vi "Add Channel to Objects.vi"(8 "error in":errorcluster, 9 "Add? (T)":bool=TRUE, 10 "Line Item in":T1, 11 "Objects in":T4) -> (0 "error out":errorcluster, 2 "Line Index":i32)   [LabVIEW 2013, in "FPGA Module editor node.lvclass"]
doc: "This VI adds the channel to the configuration Objects, and links the tag and the channel in the engine."
uses:
  FPGA Module editor node.lvclass
  <vilib>/NI/DCAF/Tag Editor Core/Table API/Table Manager/object ref.ctl
  <vilib>/NI/DCAF/Tag Editor Core/Configuration Editor/Classes/Engine Parent/Engine Parent Editor Node.lvclass
  <vilib>/NI/DCAF/Tag Editor Core/Configuration Editor/Classes/Module editor node/module editor node.lvclass
  Mappings.ctl
  <vilib>/NI/Tag Bus Module Framework/channel/TBM channel.lvclass
  module/configuration/Line.ctl
  Map.ctl
  module/configuration/FPGA Module configuration.lvclass
  <vilib>/NI/Configuration Framework/serializable configuration/NISE_CEF_serializable configuration.lvclass/NISE_CEF_serializable configuration.ctl
  <vilib>/Utility/LVClass/Get LV Class Name.vi
  <vilib>/NI/Configuration Framework/error generator/NISE_error generator.vi
  <vilib>/NI/Configuration Framework/serializable configuration/NISE_CEF_serializable configuration.lvclass
  <vilib>/NI/DCAF/Tag Editor Core/Table API/Table Manager/Table Manager.lvclass
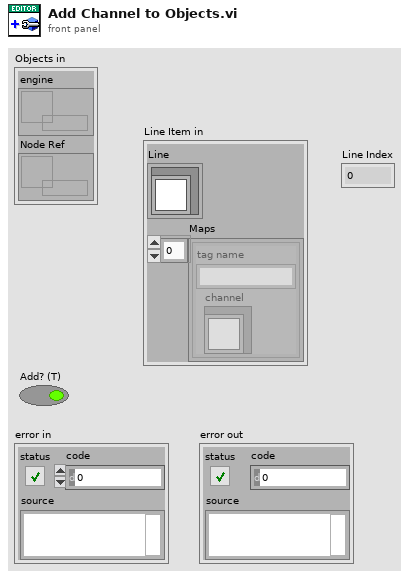
[diagram p1: front panel]
types:
  T1 = typedef "FPGA Module editor node.lvclass/Mappings.ctl" = cluster{"Line":T2, "Maps":T3[]}
  T2 = typedef "FPGA Module configuration.lvclass/Line.ctl" = cluster{"channel":refnum<class "TBM channel.lvclass">}
  T3 = typedef "FPGA Module editor node.lvclass/Map.ctl" = cluster{"channel":refnum<class "TBM channel.lvclass">, "tag name":string}
  T4 = typedef "Table Manager.lvlib/Table Manager.lvclass/object ref.ctl" = cluster{"engine":refnum<data-value>, "Node Ref":refnum<data-value>}
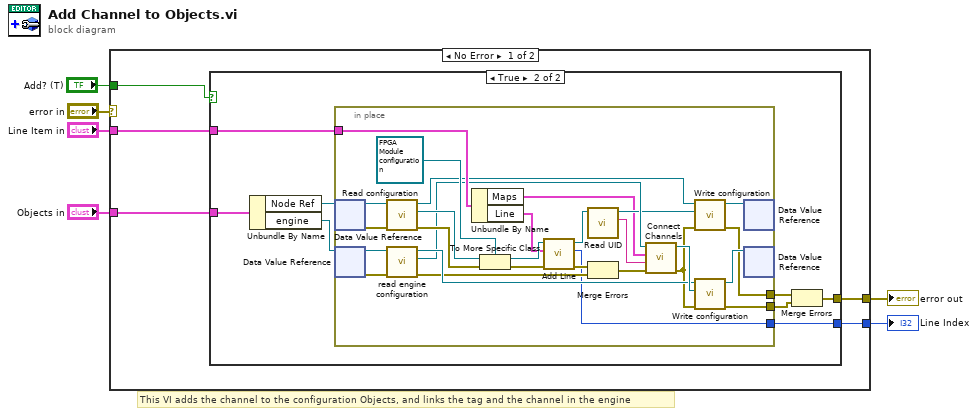
[diagram p0: block diagram]
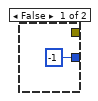
[diagram p2: hidden frame]
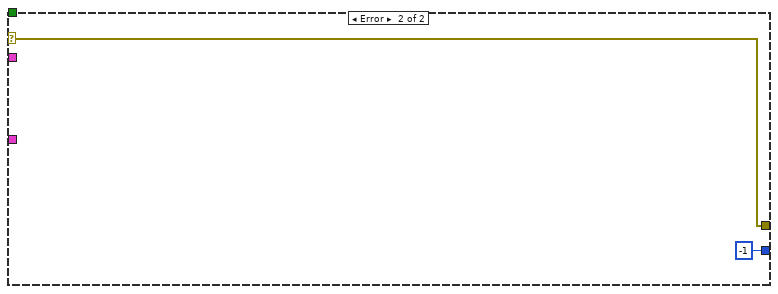
[diagram p3: hidden frame]
diagram:
  # "This VI adds the channel to the configuration Objects, and links the tag and the channel in the engine"
  n1 = case shown="No Error" "error in" {
    selector: "error in" -> [_ w50]
    tunnel: "Objects in" -> [w11 _]
    tunnel: "Line Item in" -> [w10 _]
    tunnel: "Add? (T)" -> [w9 _]
    tunnel: [w8 w50] -> w2
    tunnel: [w7 -1 ("Line Index")] -> w1
    frame No Error {
      n2 = case shown="True" w9 {
        tunnel: [_ w18] -> w8
        tunnel: w10 -> [_ w20]
        tunnel: w11 -> [_ w19]
        tunnel: [-1 ("Line Index") w13] -> w7
        frame False {
        }
        frame True {
          n3 = Unbundle By Name(w19) -> ("Node Ref"=w17:refnum<data-value>, "engine"=w16:refnum<data-value>)
          n4 = in-place {
            in-place-border: w20 -> [w48]
            in-place-border: [w35] -> w15
            in-place-border: [w33] -> w14
            in-place-border: [w21] -> w13
            n5 = in-place-dvr #1(w17) -> (w42:refnum<class "module editor node.lvclass">, w34:errorcluster)
            n6 = in-place-dvr #2(w16) -> (w32:refnum<class "Engine Parent Editor Node.lvclass">, w31:errorcluster)
            n7 = call-dynamic "Read configuration.vi"("error in"=w34, "NISE_CEF_serializable node in"=w42) -> ("error out"=w36:errorcluster, "configuration"=w37:refnum<class "NISE_CEF_serializable configuration.lvclass">, "NISE_CEF_serializable node out"=w41:refnum<class "module editor node.lvclass">)  [unwired: 7 in]
            n8 = call <vilib>:"read engine configuration.vi"("error in"=w31, "Engine Parent Editor Node in"=w32) -> ("error out"=w28:errorcluster, "engine configuration"=w29:refnum<class "engine configuration.lvclass">, "Engine Parent Editor Node out"=w30:refnum<class "Engine Parent Editor Node.lvclass">)  [unwired: 7 in]
            n9 = Unbundle By Name(w48) -> ("Maps"=w24:T3[], "Line"=w23:T2)
            n10 = To More Specific Class(target class=refnum<class "FPGA Module configuration.lvclass"> refnum ("tag bus configurable plugin module configuration in"), reference=w37, error in=w36) -> (specific class reference=w46:refnum<class "FPGA Module configuration.lvclass">, error out=w45:errorcluster)
            n11 = call "Add Line.vi"("error in"=w45, "Line"=w23, "FPGA Module configuration in"=w46) -> ("error out"=w44:errorcluster, "Line Index"=w21:i32, "FPGA Module configuration out"=w27:refnum<class "FPGA Module configuration.lvclass">)  [unwired: 6 in]
            n12 = call <vilib>:"Read UID.vi"("configuration in"=w27) -> ("instance id"=w26:string, "configuration out"=w25:refnum<class "FPGA Module configuration.lvclass">)  [unwired: 8 in, 1 out]
            n13 = Merge Errors(w44, w28) -> (w43:errorcluster)
            n14 = call "Connect Channels.vi"("error in (no error)"=w43, "instance id"=w26, "Maps"=w24, "Engine Configuration in"=w29) -> ("error out"=w22:errorcluster, "Engine Configuration out"=w38:refnum<class "engine configuration.lvclass">)  [unwired: 6 in]
            n15 = call-dynamic "Write configuration.vi"("error in"=w22, "configuration"=w25, "NISE_CEF_serializable node in"=w41) -> ("error out"=w33:errorcluster, "NISE_CEF_serializable node out"=w40:refnum<class "module editor node.lvclass">)  [unwired: 7 in]
            n16 = call-dynamic "Write configuration.vi"("error in"=w22, "configuration"=w38, "NISE_CEF_serializable node in"=w30) -> ("error out"=w35:errorcluster, "NISE_CEF_serializable node out"=w39:refnum<class "Engine Parent Editor Node.lvclass">)  [unwired: 7 in]
            n17 = in-place-dvr #1(w40) -> ()  [unwired: 2 out]
            n18 = in-place-dvr #2(w39) -> ()  [unwired: 2 out]
          }
          n19 = Merge Errors(w14, w15) -> (w18:errorcluster)
        }
      }
    }
    frame Error {
    }
  }
  "error out" <- w2
  "Line Index" <- w1
